vi "ics.vi"() -> ()   [LabVIEW 2014]
panel:
  in  "ON 15":bool
  in  "ON 14":bool
  out "Vact 15":dbl=1.0 format="%.1f"
  in  "Vset 15":dbl=1.0 format="%.1f"
  out "Vact 14":dbl=1.0 format="%.1f"
  in  "Vset 14":dbl=1.0 format="%.1f"
  in  "ON 13":bool
  in  "ON 12":bool
  out "Vact 13":dbl=1.0 format="%.1f"
  in  "Vset 13":dbl=1.0 format="%.1f"
  out "Vact 12":dbl=1.0 format="%.1f"
  in  "Vset 12":dbl=1.0 format="%.1f"
  in  "ON 7":bool
  in  "ON 6":bool
  in  "ON 5":bool
  in  "ON 4":bool
  out "Vact 7":dbl=1.0 format="%.1f"
  in  "Vset 7":dbl=1.0 format="%.1f"
  out "Vact 6":dbl=1.0 format="%.1f"
  in  "Vset 6":dbl=1.0 format="%.1f"
  out "Vact 5":dbl=1.0 format="%.1f"
  in  "Vset 5":dbl=1.0 format="%.1f"
  out "Vact 4":dbl=1.0 format="%.1f"
  in  "Vset 4":dbl=1.0 format="%.1f"
  in  "ON 11":bool
  in  "ON 10":bool
  out "Vact 11":dbl=1.0 format="%.1f"
  in  "Vset 11":dbl=1.0 format="%.1f"
  out "Vact 10":dbl=1.0 format="%.1f"
  in  "Vset 10":dbl=1.0 format="%.1f"
  in  "ON 9":bool
  in  "ON 8":bool
  in  "ON 3":bool
  in  "ON 2":bool
  in  "ON 1":bool
  in  "ON 0":bool
  out "Vact 3":dbl=1.0 format="%.1f"
  in  "Vset 3":dbl=1.0 format="%.1f"
  out "Vact 2":dbl=1.0 format="%.1f"
  in  "Vset 2":dbl=1.0 format="%.1f"
  in  "Steps 1":i32
  in  "Config 1":string="{8:1,9:-1}"
  in  "Steps 0":i32
  in  "Config 0":string="{8:1,9:1}"
  out "Vact 9":dbl=1.0 format="%.1f"
  in  "Vset 9":dbl=1.0 format="%.1f"
  out "Vact 8":dbl=1.0 format="%.1f"
  in  "Vset 8":dbl=1.0 format="%.1f"
  out "Vact 1":dbl=1.0 format="%.1f"
  in  "Vset 1":dbl=1.0 format="%.1f"
  out "Vact 0":dbl=1.0 format="%.1f"
  in  "Vset 0":dbl=1.0 format="%.1f"
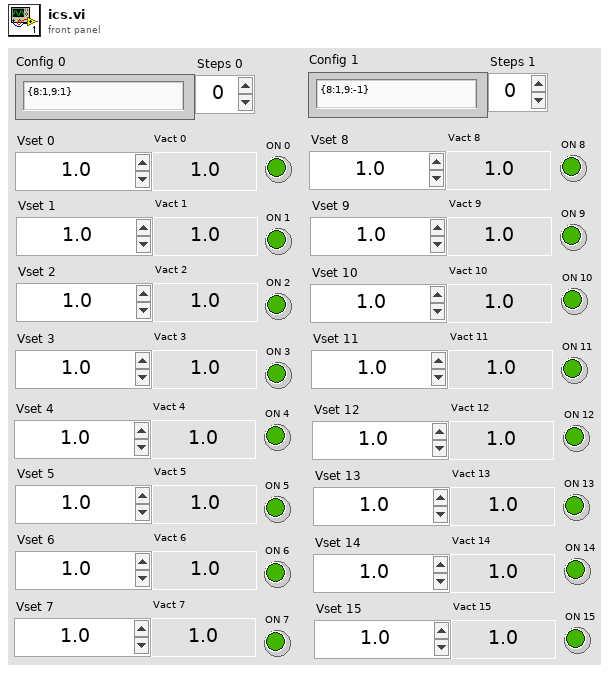
[diagram p1: front panel]
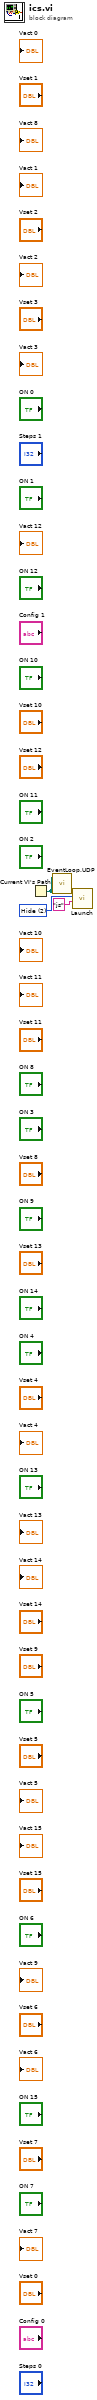
[diagram p0: block diagram]
diagram:
  w1 = u16 2 items=["Normal", "Keep", "Hide"] ("Mode")
  n1 = Current VI's Path() -> (path=w3:path)
  n2 = call "EventLoop.UDP.vi"("Path"=w3) -> ()  [unwired: 2 in]
  n3 = call "Launch.vi"("Cmd"="js", "Mode"=w1, "Path"=w3) -> ()  [unwired: 1 in]
